vi "Indexer.vi"(8 "error in (no error)":errorcluster, 11 "Robot Commands":T1) -> (0 "error out":errorcluster)   [LabVIEW 2015]
uses:
  Joystick/Robot Commands.ctl
  <vilib>/Rock Robotics/WPI/Relay/WPI_RelayValue.ctl
  Global Variables/Refnum Names.vi
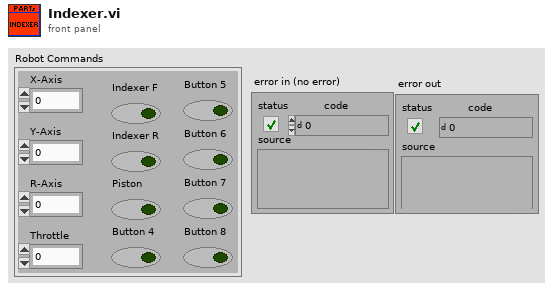
[diagram p1: front panel]
types:
  T1 = typedef "Robot Commands.ctl" = cluster{"X-Axis":dbl, "Y-Axis":dbl, "R-Axis":dbl, "Throttle":dbl, "Indexer F":bool, "Indexer R":bool, "Piston":bool, "Button 4":bool, "Button 5":bool, "Button 6":bool, "Button 7":bool, "Button 8":bool}
  T2 = typedef "WPI_RelayValue.ctl" = enum16{"Off", "On", "Forward", "Reverse"}
  T3 = typedef "WPI_RelayDevRef.ctl" = cluster{"DevStatus":errorcluster, "Relay Channel":T4, "Relay Direction":T5}
  T4 = typedef "FPGA_DIORelayChannel.ctl" = enum8{"Relay 0", "Relay 1", "Relay 2", "Relay 3", "Invalid"}
  T5 = typedef "WPI_RelayDirection.ctl" = enum16{"Both directions", "Forward only", "Reverse only"}
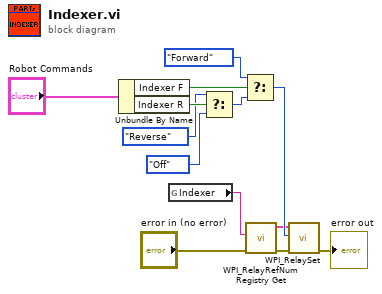
[diagram p0: block diagram]
diagram:
  n1 = Unbundle By Name("Robot Commands") -> ("Indexer F"=w8:bool, "Indexer R"=w6:bool)
  n2 = global read "Refnum Names.vi" "Indexer"() -> (w13:string)
  n3 = Select(t=WPI_RelayValue."Reverse" ("RelayValue"), s=w6, f=WPI_RelayValue."Off" ("RelayValue")) -> (s? t:f=w4:T2)
  n4 = Select(t=WPI_RelayValue."Forward" ("RelayValue"), s=w8, f=w4) -> (s? t:f=w12:T2)
  n5 = call <vilib>:"WPI_RelayRefNum Registry Get.vi"("error in (no error)"="error in (no error)", "refnum name"=w13) -> ("error out"=w11:errorcluster, "RelayDevRef"=w10:T3)  [unwired: 8 in]
  n6 = call <vilib>:"WPI_RelaySet.vi"("error in (no error)"=w11, "RelayValue"=w12, "RelayDevRef"=w10) -> ("error out"=→"error out":errorcluster)  [unwired: 7 in, 1 out]
